vi "SO2 Calibration Equation.vi"(0 "Input":dbl, 7 "Offset":dbl, 11 "Slope":dbl) -> (8 "Output":dbl)   [LabVIEW 2014]
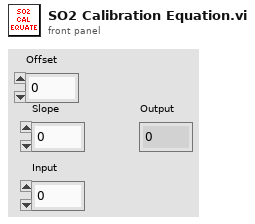
[diagram p1: front panel]
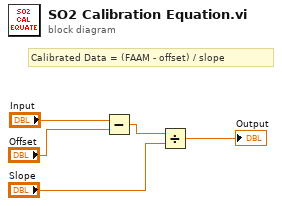
[diagram p0: block diagram]
diagram:
  # "Calibrated Data = (FAAM - offset) / slope"
  n1 = Subtract(x="Input", y="Offset") -> (x-y=w3:dbl)
  n2 = Divide(x=w3, y="Slope") -> (x/y=→"Output":dbl)
